vi "Read Cal On.vi"(8 "error in (no error)":errorcluster, 11 "Pressure Calibration Command in":refnum<class "Pressure Calibration Command.lvclass">) -> (0 "error out":errorcluster, 2 "Cal On?":bool, 3 "Pressure Calibration Command out":refnum<class "Pressure Calibration Command.lvclass">)   [LabVIEW 2014, in "Pressure Calibration Command.lvclass"]
uses:
  Pressure Calibration Command.lvclass
  Pressure Calibration Command.lvclass/Pressure Calibration Command.ctl
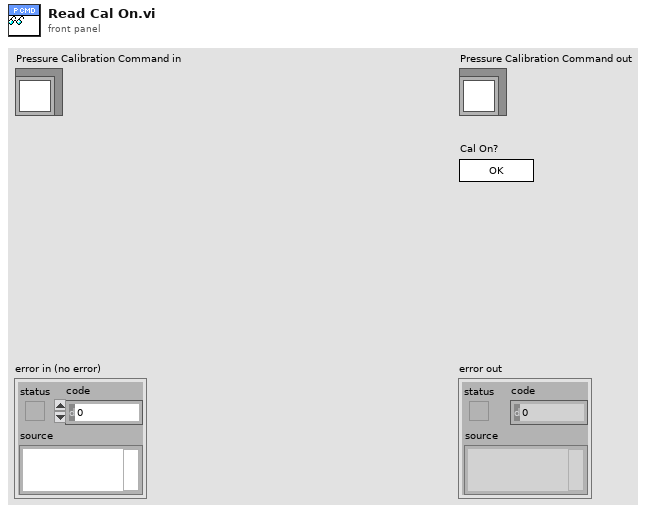
[diagram p1: front panel]
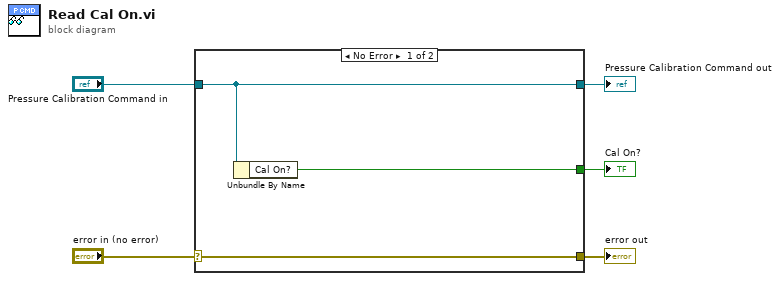
[diagram p0: block diagram]
diagram:
  n1 = case shown="No Error" "error in (no error)" {
    selector: "error in (no error)" -> [w8 w9]
    tunnel: [w8 w9] -> w4
    tunnel: [w7 w10] -> w2
    tunnel: "Pressure Calibration Command in" -> [w7 w10]
    tunnel: [w6 _] -> w1
    frame No Error {
      n2 = Unbundle By Name(w7) -> ("Cal On?"=w6:bool)
    }
    frame Error {
    }
  }
  "error out" <- w4
  "Pressure Calibration Command out" <- w2
  "Cal On?" <- w1
